vi "Setpoint Generation.vi"(1 "Setpoint":T1) -> (0 "Setpoint signal output":dbl[](array[numeric]))   [LabVIEW 2018]
uses:
  Host/controls/Setpoints.ctl
  <vilib>/ptbypt/NI_PtbyPt.lvlib
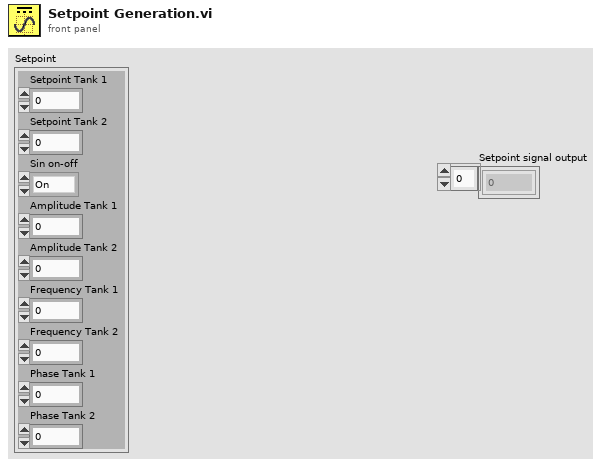
[diagram p1: front panel]
types:
  T1 = typedef "Setpoints.ctl" = cluster{"Setpoint Tank 1":dbl, "Setpoint Tank 2":dbl, "Sin on-off":enum32{"On", "Off"}, "Amplitude Tank 1":dbl, "Amplitude Tank 2":dbl, "Frequency Tank 1":dbl, "Frequency Tank 2":dbl, "Phase Tank 1":dbl, "Phase Tank 2":dbl}
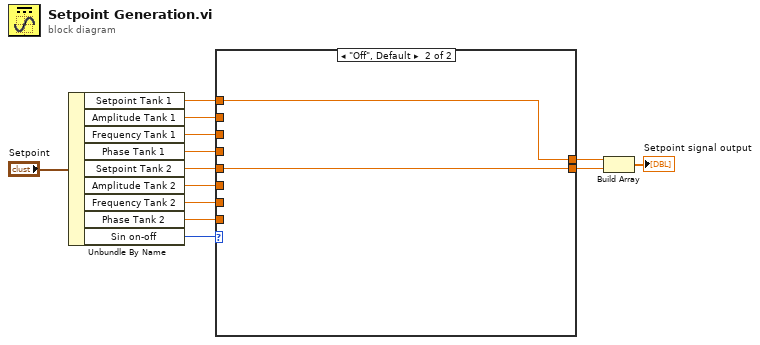
[diagram p0: block diagram]
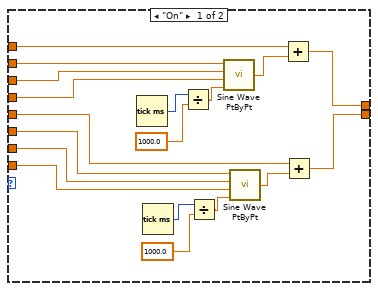
[diagram p2: hidden frame]
diagram:
  n1 = Unbundle By Name("Setpoint") -> ("Setpoint Tank 1"=w6:dbl, "Amplitude Tank 1"=w7:dbl, "Frequency Tank 1"=w8:dbl, "Phase Tank 1"=w9:dbl, "Setpoint Tank 2"=w10:dbl, "Amplitude Tank 2"=w11:dbl, "Frequency Tank 2"=w12:dbl, "Phase Tank 2"=w13:dbl, "Sin on-off"=w5:enum32{"On", "Off"})
  n2 = case shown="\"Off\", Default" w5 {
    tunnel: w6 -> [w16 w33]
    tunnel: w7 -> [w25 _]
    tunnel: w8 -> [w24 _]
    tunnel: w9 -> [w23 _]
    tunnel: w10 -> [w18 w32]
    tunnel: w11 -> [w22 _]
    tunnel: w12 -> [w21 _]
    tunnel: w13 -> [w20 _]
    tunnel: [w15 w33] -> w3
    tunnel: [w14 w32] -> w2
    frame "On" {
      n3 = Tick Count (ms)() -> (millisecond timer value=w28:u32)
      n4 = Tick Count (ms)() -> (millisecond timer value=w29:u32)
      n5 = Divide(x=w28, y=1000.0 ("x")) -> (x/y=w26:dbl)
      n6 = Divide(x=w29, y=1000.0 ("x")) -> (x/y=w31:dbl)
      n7 = call <vilib>:"Sine Wave PtByPt.vi"("time"=w26, "phase"=w23, "frequency"=w24, "amplitude"=w25) -> ("sine wave"=w17:dbl)
      n8 = call <vilib>:"Sine Wave PtByPt.vi"("time"=w31, "phase"=w20, "frequency"=w21, "amplitude"=w22) -> ("sine wave"=w19:dbl)
      n9 = Add(x=w16, y=w17) -> (x+y=w15:dbl)
      n10 = Add(x=w18, y=w19) -> (x+y=w14:dbl)
    }
    frame "Off", Default {
    }
  }
  n11 = Build Array(w3, w2) -> (→"Setpoint signal output":dbl[])
